vi "currently listening.vi"(11 "TCP server in":refnum<class "TCP server.lvclass">) -> (3 "listening?":bool)   [LabVIEW 2015, in "TCP server.lvclass"]
uses:
  TCP server.lvclass
  TCP server.lvclass/TCP server.ctl
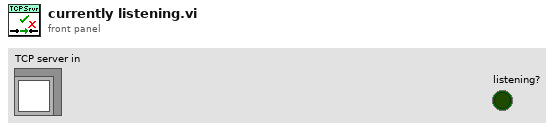
[diagram p1: front panel]
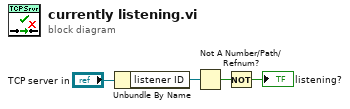
[diagram p0: block diagram]
diagram:
  n1 = Unbundle By Name("TCP server in") -> ("listener ID"=w3:refnum<k5>)
  n2 = Not A Number/Path/Refnum?(number/path/refnum=w3) -> (NaN/Path/Refnum?=w2:bool)
  n3 = Not(x=w2) -> (.not. x?=→"listening?":bool)
